vi "Venturi.vi"(8 "T":dbl, 9 "A1/A2":dbl, 10 "P":dbl, 11 "V":dbl) -> (0 "V2":dbl, 1 "Density":dbl[unit], 2 "P2":dbl, 3 "dPventury":dbl[unit])   [LabVIEW 2019]
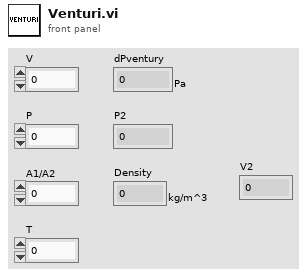
[diagram p1: front panel]
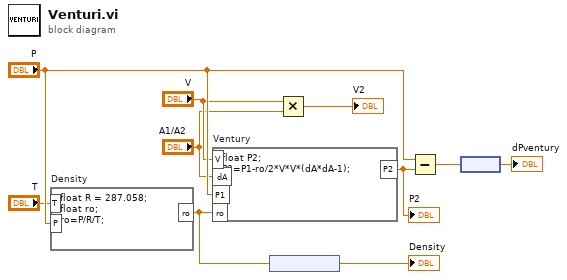
[diagram p0: block diagram]
diagram:
  n1 = formula code="float R = 287.058;\nfloat ro;\nro=P/R/T;" "Density"("P"="P", "T"="T") -> ("ro"=w6:dbl)
  n2 = formula code="float P2;\nP2=P1-ro/2*V*V*(dA*dA-1);" "Ventury"("dA"="A1/A2", "P1"="P", "V"="V", "ro"=w6) -> ("P2"=w8:dbl)
  "P2" <- w8
  n3 = node(w6) -> (→"Density":dbl[unit])
  n4 = Multiply(x="V", y="A1/A2") -> (x*y=→"V2":dbl)
  n5 = Subtract(x="P", y=w8) -> (x-y=w9:dbl)
  n6 = node(w9) -> (→"dPventury":dbl[unit])
